vi "SetAttributeViBoolean_SA-Gating_Sweep.vi"(7 "AttributeValue (Off)":bool, 8 "error in (no error)":errorcluster {"code" format="%.0x"}, 9 "AttributeID":u32(ring)=1150527 items=["SA_GATING_ENABLED"=1150527, "SA_GATING_HOLD_OFF_TIME_AUTO_ENABLED"=1150536, "SA_GATING_VIEW"=1150533, "SA_LISTSWEEP_ENABLED"=1150754, "SA_LISTSWEEP_FREQUENCY_SYNTHESIS_AUTO_ENABLED"=1150640, "SA_LISTSWEEP_SEQUENCE_AUTO_ENABLED"=1150642, "SA_SWEEPCOUPLING_BANDWIDTH_RATIO_AUTO_ENABLED"=1150723, "SA_SWEEPCOUPLING_FFT_WIDTH_AUTO_ENABLED"=1150726, "SA_SWEEPCOUPLING_SWEEP_TIME_AUTO_RULES_AUTO_ENABLED"=1150733, "SA_SWEEPCOUPLING_SWEEP_TYPE_AUTO_ENABLED"=1150735, "SA_SWEEPCOUPLING_SWEEP_TYPE_AUTO_RULES_AUTO_ENABLED"=1150729], 11 "instrument handle":refnum<k15>) -> (0 "error out":errorcluster {"code" format="%.0x"}, 3 "instrument handle out":refnum<k15>)   [LabVIEW 2009, in "Keysight XSAn.lvlib"]
doc: "Sets a Boolean attribute from the instrument driver.\nThe following Attributes are supported:\n\nSA_GATING_ENABLED\nSA_GATING_HOLD_OFF_TIME_AUTO_ENABLED\nSA_GATING_VIEW\nSA_LISTSWEEP_ENABLED\nSA_LISTSWEEP_FREQUENCY_SYNTHESIS_AUTO_ENABLED\nSA_LISTSWEEP_SEQUENCE_AUTO_ENABLED\nSA_SWEEPCOUPLING_BANDWIDTH_RATIO_AUTO_ENABLED\nSA_SWEEPCOUPLING_FFT_WIDTH_AUTO_ENABLED\nSA_SWEEPCOUPLING_SWEEP_TIME_AUTO_RULES_AUTO_ENABLED\nSA_SWEEPCOUPLING_SWEEP_TYPE_AUTO_ENABLED\nSA_SWEEPCOUPLING_SWEEP_TYPE_AUTO_RULES_AUTO_ENABLED"
uses:
  <instrlib>/Keysight XSAn/Keysight XSAn.lvlib
  AgXSAn.dll
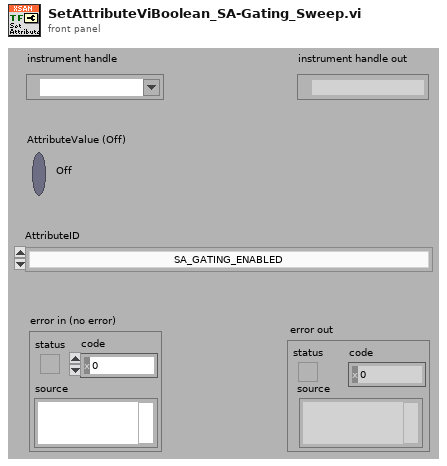
[diagram p1: front panel]
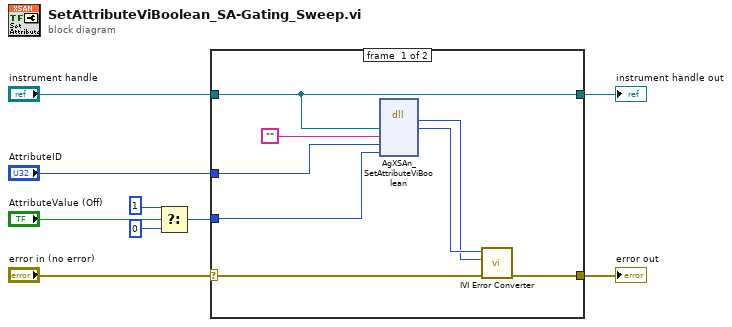
[diagram p0: block diagram]
diagram:
  n1 = Select(t=u16 1, s="AttributeValue (Off)", f=u16 0) -> (s? t:f=w2:u16)
  n2 = case shown="No Error" "error in (no error)" {
    selector: "error in (no error)" -> [w15 w19]
    tunnel: [w14 w19] -> w9
    tunnel: "instrument handle" -> [w11 w18]
    tunnel: "AttributeID" -> [w13 _]
    tunnel: w2 -> [w12 _]
    tunnel: [w11 w18] -> w1
    frame #0 {
      n3 = dll-call lib="AgXSAn**.dll" fn="AgXSAn_SetAttributeViBoolean"("Vi"=w11, "RepCapIdentifier"="", "AttributeID"=w13, "AttributeValue"=w12) -> ("return type"=w16:i32, "Vi"=w17:u32)  [unwired: 6 in, 2 out]
      n4 = call <instrlib>:"IVI Error Converter.vi"("error in (no error)"=w15, "IVI error code (0)"=w16, "instrument handle"=w17) -> ("error out"=w14:errorcluster)  [unwired: 7 in, 1 out]
    }
    frame #1 {
    }
  }
  "error out" <- w9
  "instrument handle out" <- w1
